vi "High_Power_CH1.vi"(8 "Modulation parameter":T1, 9 "output bits":i8[](array[numeric]), 10 "Boolean":bool, 11 "Record BER":bool) -> ()   [LabVIEW 2022 SP3]
panel:
  out "No. Bits LP":dbl
  out "?":T1
  out "Low-Power Decoded Message":string
  in  "Expected message LP":string="Non Critical Data\nNon Critical Data\nNon Critical Data\nNon Critical Data\nNon Critical Data"
  out "Acum. Err LP":dbl
  out "Acc. BER LP":dbl format="%#_4g"
  out "Inst. BER LP":dbl format="%#_4g"
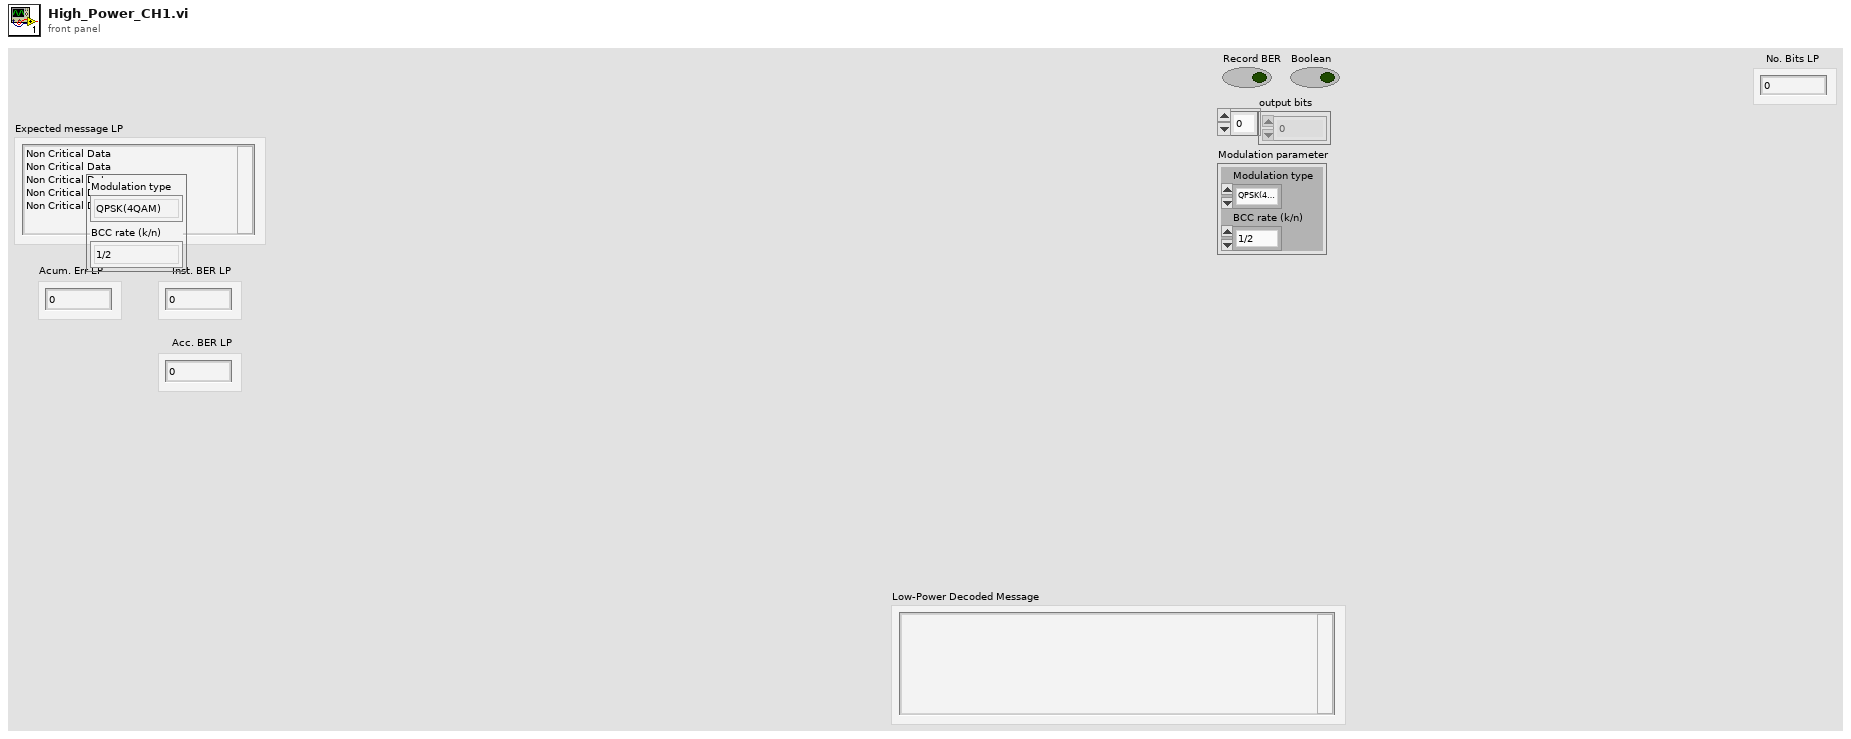
[diagram p1: front panel]
types:
  T1 = cluster{"Modulation type":enum16{"QPSK(4QAM)", "64QAM", "16QAM", "BPSK"}, "BCC rate (k/n)":enum16{"1/2", "2/3", "3/4"}}
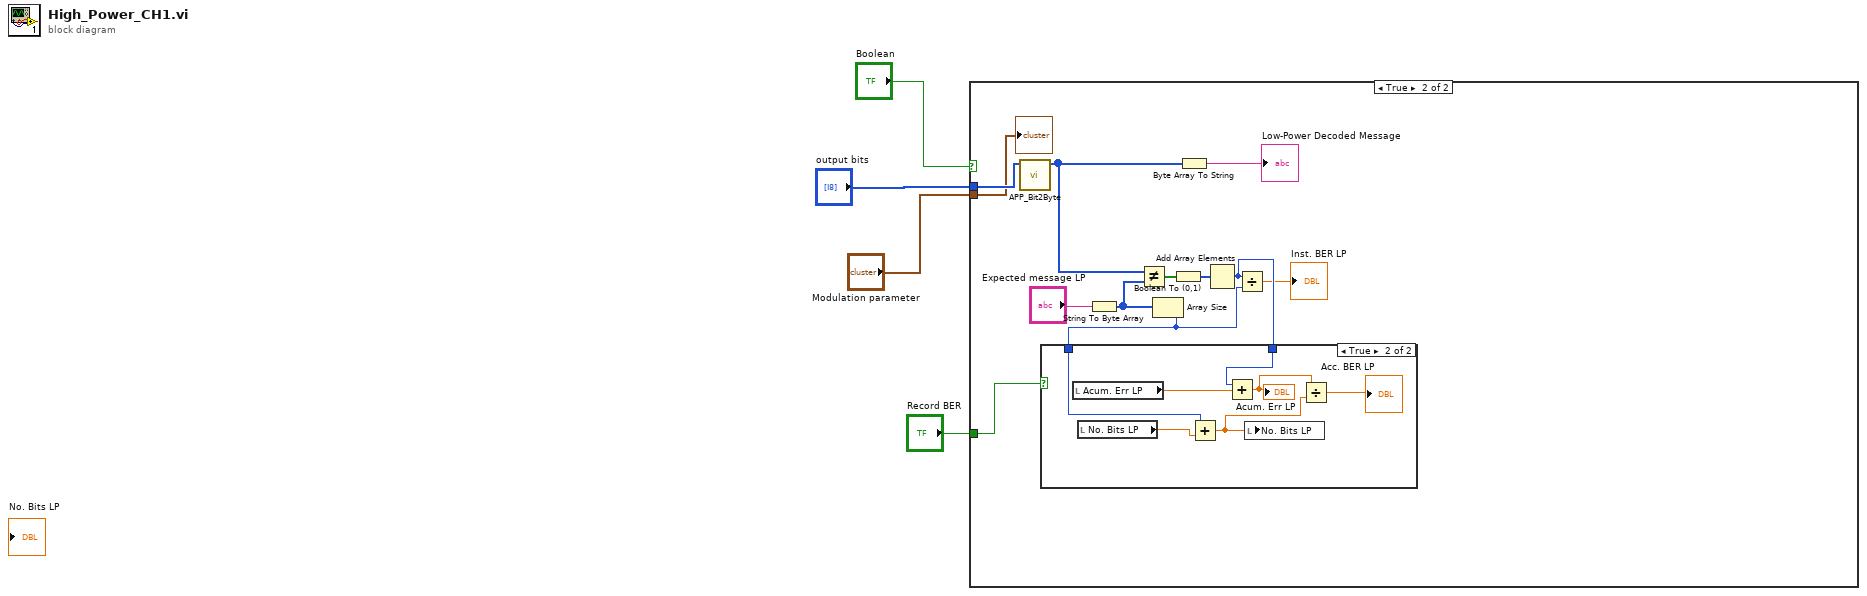
[diagram p0: block diagram]
diagram:
  n1 = case shown="True" "Boolean" {
    tunnel: "output bits" -> [_ w16]
    tunnel: "Modulation parameter" -> [_ w15]
    tunnel: "Record BER" -> [_ w6]
    frame False {
    }
    frame True {
      n2 = call "APP_Bit2Byte.vi"("input bit stream"=w16) -> ("output byte stream"=w8:u8[])  [unwired: 10 in]
      n3 = String To Byte Array(string="Expected message LP") -> (unsigned byte array=w12:u8[])
      n4 = Not Equal?(x=w8, y=w12) -> (x != y?=w10:bool[])
      n5 = Array Size(array=w12) -> (size(s)=w13:i32)
      n6 = Boolean To (0,1)(Boolean=w10) -> (0, 1=w9:i16[])
      n7 = Byte Array To String(unsigned byte array=w8) -> (string=→"Low-Power Decoded Message":string)
      n8 = Add Array Elements(numeric array=w9) -> (sum=w7:i16)
      n9 = case shown="True" w6 {
        tunnel: w13 -> [_ w22]
        tunnel: w7 -> [_ w20]
        frame False {
        }
        frame True {
          n10 = local read "Acum. Err LP"() -> (w21:dbl)
          n11 = local read "No. Bits LP"() -> (w23:dbl)
          n12 = Add(x=w22, y=w23) -> (x+y=w17:dbl)
          n13 = Add(x=w20, y=w21) -> (x+y=w19:dbl)
          "Acum. Err LP" <- w19
          n14 = local write "No. Bits LP"(w17) -> ()
          n15 = Divide(x=w19, y=w17) -> (x/y=→"Acc. BER LP":dbl)
        }
      }
      n16 = Divide(x=w7, y=w13) -> (x/y=→"Inst. BER LP":dbl)
      "?" <- w15
    }
  }
